vi "Analog Trigger Config.vi"(0 "Session Handle in":T4, 7 "Trigger Config":T1={"Channel"=enum."chn B", "Edge"=0, "Level[V]"=0.5} {"Edge" items=["RISING", "FALLING", "ANY"]}, 11 "error in (no error)":errorcluster) -> (4 "Session Handle out":T4, 15 "error out":errorcluster)   [LabVIEW 2019, in "SmartScopeDriver.lvclass"]
doc: "Configures the analog trigger for one channel."
uses:
  SmartScopeDriver.lvclass
  Typedefs/Session Handle.ctl
  Scope Driver/Typedef/TriggerData.ctl
  Scope Driver/Typedef/Channel Selection.ctl
  Scope Driver/Typedef/Edge.ctl
  SmartScopeDriver.lvclass/SmartScopeDriver.ctl
  Scope Driver/LabNation Scope Driver.lvlib
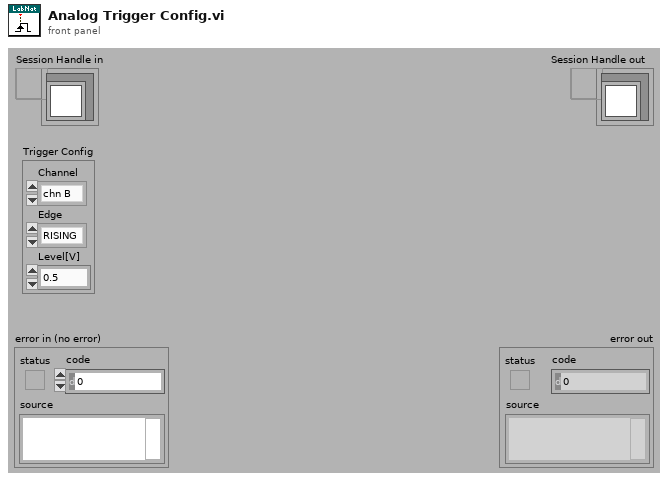
[diagram p1: front panel]
types:
  T1 = typedef "LabNation Scope Driver.lvlib/TriggerData.ctl" = cluster{"Channel":T2, "Edge":T3, "Level[V]":sgl}
  T2 = typedef "LabNation Scope Driver.lvlib/Channel Selection.ctl" = enum16{"chn A", "chn B"}
  T3 = typedef "LabNation Scope Driver.lvlib/Edge.ctl" = i32
  T4 = typedef "SmartScopeDriver.lvclass/Session Handle.ctl" = refnum<data-value>
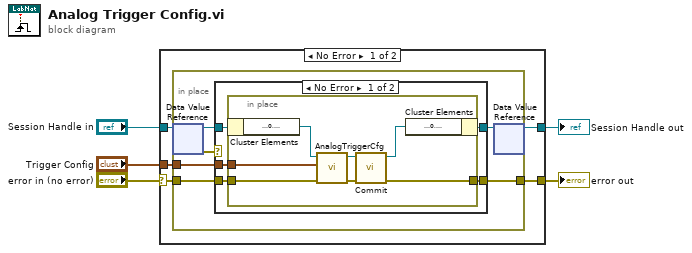
[diagram p0: block diagram]
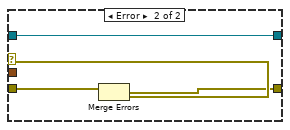
[diagram p2: hidden frame]
diagram:
  n1 = case shown="No Error" "error in (no error)" {
    selector: "error in (no error)" -> [w8 w33]
    tunnel: "Session Handle in" -> [w10 w34]
    tunnel: [w9 w34] -> w4
    tunnel: [w7 w33] -> w3
    tunnel: "Trigger Config" -> [w6 _]
    frame No Error {
      n2 = in-place {
        in-place-border: w8 -> [w12]
        in-place-border: [w15] -> w7
        in-place-border: w6 -> [w11]
        n3 = in-place-dvr #1(w10) -> (w16:refnum<class "SmartScopeDriver.lvclass">, w13:errorcluster)
        n4 = case shown="No Error" w13 {
          selector: w13 -> [_ w31]
          tunnel: w16 -> [w21 w29]
          tunnel: [w20 w30] -> w15
          tunnel: [w19 w29] -> w14
          tunnel: w12 -> [w18 w32]
          tunnel: w11 -> [w17 _]
          frame No Error {
            n5 = in-place {
              in-place-border: [w23] -> w20
              in-place-border: w18 -> [w26]
              in-place-border: w17 -> [w28]
              n6 = in-place-cluster #2(w21) -> ("reference"=w27:refnum<k24>)
              n7 = call "AnalogTriggerCfg.vi"("error in (no error)"=w26, "Trigger Config"=w28, "reference in"=w27) -> ("error out"=w24:errorcluster, "reference out"=w25:refnum<k24>)  [unwired: 7 in]
              n8 = call "Commit.vi"("error in (no error)"=w24, "reference in"=w25) -> ("error out"=w23:errorcluster, "reference out"=w22:refnum<k24>)  [unwired: 8 in]
              n9 = in-place-cluster #2("reference"=w22) -> (w19:refnum<class "SmartScopeDriver.lvclass">)
            }
          }
          frame Error {
            n10 = Merge Errors(w32, w31) -> (w30:errorcluster)
          }
        }
        n11 = in-place-dvr #1(w14) -> (w9:T4)  [unwired: 1 out]
      }
    }
    frame Error {
    }
  }
  "Session Handle out" <- w4
  "error out" <- w3
